vi "lcd(suvi).vi"(7 "number":u8[](array[numeric]), 8 "error in (no error)":errorcluster, 9 "String":string, 10 "location":u8[](array[numeric]), 11 "LINX Resource in":T1) -> (0 "error out":errorcluster, 1 "LINX Resource":T1, 2 "number out":u8[](array[numeric]), 3 "string out":string)   [LabVIEW 2020]
uses:
  <vilib>/MakerHub/LINX/Private/Type Defs/LINX Ref.ctl
  <vilib>/MakerHub/LINX/Private/Type Defs/Platform.ctl
  <vilib>/MakerHub/LINX/Private/Type Defs/Interface.ctl
  <vilib>/MakerHub/LINX/Private/Device/Type Defs/LINX Device Config.ctl
  <vilib>/MakerHub/LINX/Private/Device/Type Defs/TCP Config.ctl
  <vilib>/MakerHub/LINX/Private/Device/Type Defs/Channels.ctl
  <vilib>/MakerHub/LINX/LMH-LINX.lvlib
  <vilib>/MakerHub/LINX/Private/Device/Device.lvlib
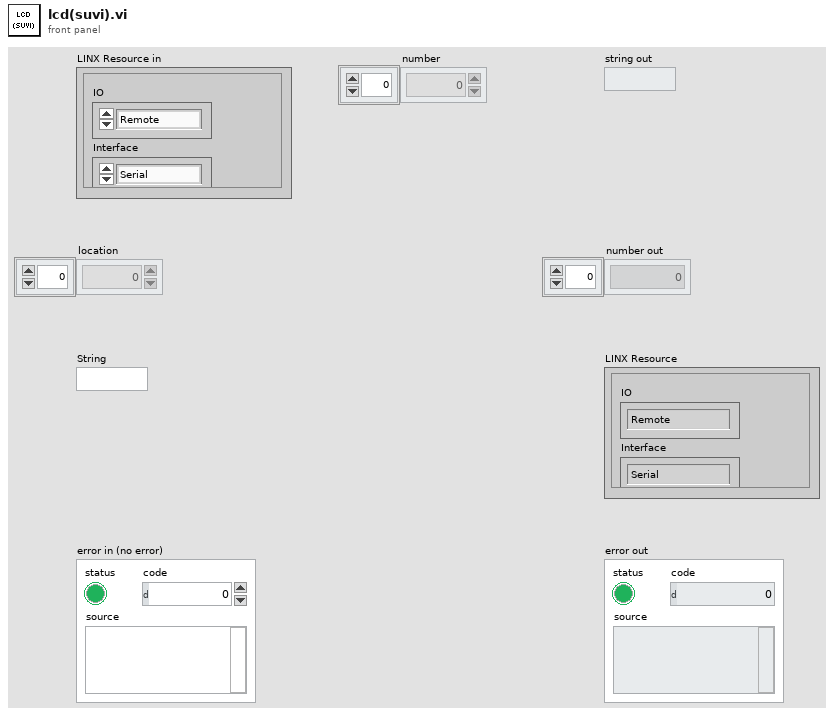
[diagram p1: front panel]
types:
  T1 = typedef "LMH-LINX.lvlib/LINX Ref.ctl" = cluster{"IO":T2, "Interface":T3, "LINX Device Config":T4}
  T2 = typedef "LMH-LINX.lvlib/Platform.ctl" = enum16{"Remote", "Local"}
  T3 = typedef "LMH-LINX.lvlib/Interface.ctl" = enum16{"Serial", "TCP"}
  T4 = typedef "LMH-LINX.lvlib/Device.lvlib/LINX Device Config.ctl" = cluster{"Interface":T3, "COM Port":refnum<visa-resource-name>, "TCP Configuration":T5, "Device Family":u8, "Device ID":u8, "Device Name":string, "TCP Ref":refnum<k5>, "Channels":T6}
  T5 = typedef "LMH-LINX.lvlib/Device.lvlib/TCP Config.ctl" = cluster{"IP Address":string, "Port":u16}
  T6 = typedef "LMH-LINX.lvlib/Channels.ctl" = cluster{"DI":u8[], "DO":u8[], "AI":u8[], "AO":u8[], "PWM":u8[], "QE":u8[], "UART":u8[], "I2C 2":u8[], "SPI":u8[], "CAN":u8[], "Servo":u8[], "AI Ref (V)":dbl, "AI Resolution (Bits)":u8, "AO Ref (V)":dbl, "AO Resolution (Bits)":u8}
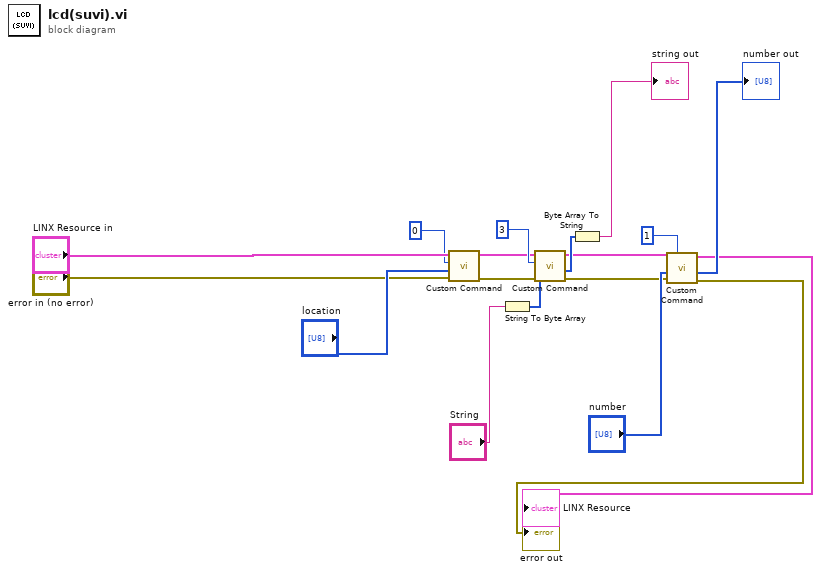
[diagram p0: block diagram]
diagram:
  n1 = call <vilib>:"Custom Command.vi"("Error In"="error in (no error)", "Data"="location", "Custom Command Number"=u16 0, "LINX Resource"="LINX Resource in") -> ("Error Out"=w5:errorcluster, "LINX Resource"=w7:T1)  [unwired: 4 in, 2 out]
  n2 = String To Byte Array(string="String") -> (unsigned byte array=w13:u8[])
  n3 = call <vilib>:"Custom Command.vi"("Error In"=w5, "Data"=w13, "Custom Command Number"=u16 3, "LINX Resource"=w7) -> ("Error Out"=w3:errorcluster, "Response"=w12:u8[], "LINX Resource"=w4:T1)  [unwired: 4 in, 1 out]
  n4 = Byte Array To String(unsigned byte array=w12) -> (string=→"string out":string)
  n5 = call <vilib>:"Custom Command.vi"("Error In"=w3, "Data"="number", "Custom Command Number"=u16 1, "LINX Resource"=w4) -> ("Error Out"=→"error out":errorcluster, "Response"=→"number out":u8[], "LINX Resource"=→"LINX Resource":T1)  [unwired: 4 in, 1 out]
